vi "SS_observer_Delay.vi"(4 "Xd_in":T1=[0.0, 0.0, 0.0, 0.0, 0.0, 0.0, 0.0, 0.0, 0.0, 0.0, 0.0, 0.0] caption="Xd_In", 7 "y(k)":sgl format="%#_13g", 8 "Nd":u8, 9 "X":sgl[](array[numeric])=[0.0, 0.0, 0.0, 0.0, 0.0, 0.0, 0.0, 0.0, 0.0, 0.0, 0.0, 0.0, 0.0, 0.0, 0.0, 0.0, 0.0, 0.0, 0.0, 0.0, 0.0, 0.0, 0.0, 0.0, 0.0], 10 "u(predelay)(k)":sgl format="%#_13g", 11 "NS":i16) -> (3 "Ax + Bu + Lye":sgl[](array[numeric]), 6 "Xd_out":T1)   [LabVIEW 2017]
uses:
  controls/Xdelay.ctl
  <vilib>/Platform/TimedLoop/XDataNode/timing_clust.ctl
  <vilib>/Platform/TimedLoop/XDataNode/nitl_modes.ctl
  <vilib>/Platform/TimedLoop/XDataNode/wakeup.ctl
  <vilib>/rvi/Emulation/niFpgaSctlEmulationGetInTimedLoop.vi
  <vilib>/rvi/Emulation/niFpgaEmulationReportErrorSimple.vi
  <vilib>/rvi/Emulation/niFpgaGetClockAttributes.vi
  <vilib>/rvi/Emulation/niFpgaCriticalErrorInLSC.vi
  <vilib>/Platform/TimedLoop/XDataNode/XDataNode.xnode
  <vilib>/Platform/TimedLoop/XDataNode/XDNodeRunTimeDep.lvlib
panel:
  out "u(k)":sgl format="%#_13g"
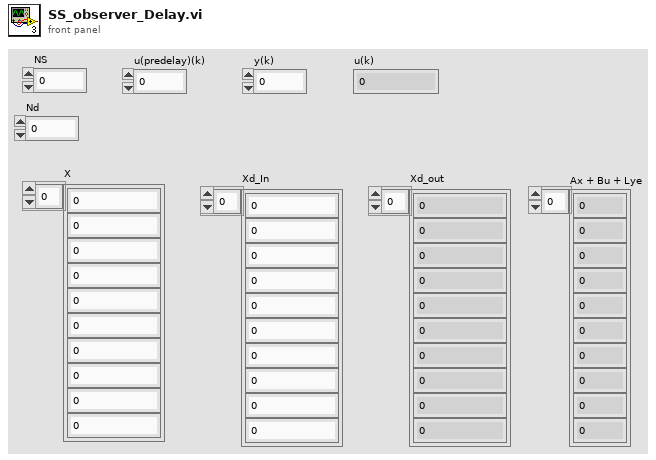
[diagram p1: front panel]
types:
  T1 = typedef "Xdelay.ctl" = sgl[]
  T2 = typedef "XDNodeRunTimeDep.lvlib/timing_clust.ctl" = cluster{"Expected End [f-1]":u64, "Actual End [f-1]":u64, "Finished Late? [f-1]":bool, "Expected End [i-1]":u64, "Actual End [i-1]":u64, "Finished Late? [i-1]":bool, "Expected Start [i]":u64, "Actual Start [i]":u64, "Expected Start [f]":u64, "Actual Start [f]":u64, "Source Name":string, "Structure Name":string, "Period":i64, "Deadline":i64, "Offset":i64, "Start":i64, "Priority":i32, "Timeout":i32, "Mode":T3, "Wakeup Reason":T4, "Error":errorcluster, "Source Type":string, "Secondary Source Type":string, "Global End Time":u64, "Global Start Time":u64, "Frame Duration":u64, "Iteration Duration":u64, "Assigned CPU":i32, "I/O Scan Engine Mode":u32}
  T3 = typedef "XDNodeRunTimeDep.lvlib/nitl_modes.ctl" = enum32{"No Change", "Process missed periods, maintain original phase", "Discard missed periods, maintain original phase", "Process missed periods, ignore original phase", "Discard missed periods, ignore original phase"}
  T4 = typedef "XDNodeRunTimeDep.lvlib/wakeup.ctl" = enum32{"Normal", "Aborted", "Asynchronous wakeup", "Timing source error", "Timed loop error", "Timeout"}
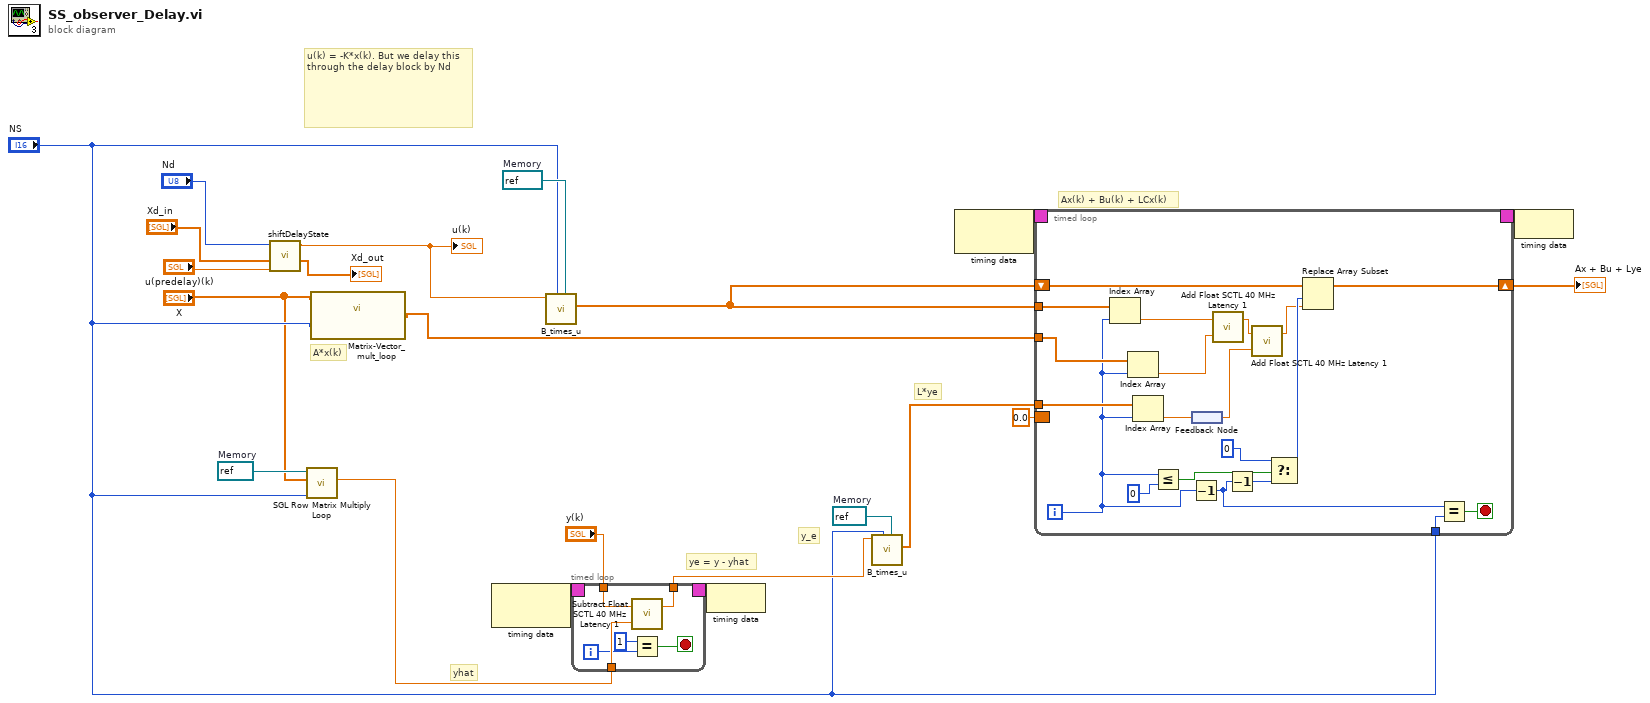
[diagram p0: block diagram]
diagram:
  w16 = refnum<k21> "L"  # Memory
  w15 = refnum<k21> "C"  # Memory
  w14 = refnum<k21> "Bz"  # Memory
  # "ye = y - yhat"
  # "yhat"
  # "A*x(k)"
  # "L*ye"
  # "y_e"
  # "u(k) = -K*x(k). But we delay this through the delay block by Nd"
  # "Ax(k) + Bu(k) + LCx(k)"
  n1 = call "shiftDelayState.vi"("u(k)"="u(predelay)(k)", "Xd_in"="Xd_in", "Nd"="Nd") -> ("Xd_out"=→"Xd_out":T1, "yd=C*Xd(k)"=w8:sgl)  [unwired: 7 in]
  "u(k)" <- w8
  n2 = call "SGL Row Matrix Multiply Loop.vi"("NS"="NS", "X"="X", "Refnum in"=w15) -> ("Numeric"=w12:sgl)  [unwired: 8 in]
  n3 = call "Matrix-Vector_mult_loop.vi"("Ns"="NS", "X"="X") -> ("A x X"=w3:sgl[])  [unwired: 9 in]
  n4 = node-c288() -> (w20:T2)  [unwired: 1 in]
  n5 = call "B_times_u.vi"("Memory"=w14, "NS"="NS", "u"=w8) -> ("product(vector)"=w9:sgl[])  [unwired: 8 in]
  n6 = timed-loop {
    timing: w20 -> [_]
    timing-out: [_] -> w19
    tunnel: [w28] -> w10
    tunnel: "y(k)" -> [w27]
    tunnel: w12 -> [w26]
    i -> [w24]
    stop <- w25 stop-if-true
    n7 = call "Subtract Float SCTL 40 MHz Latency 1.vi"("y"=w26, "x"=w27) -> ("x[k-1]-y[k-1]"=w28:sgl)  [unwired: 1 out]
    n8 = Equal?(x=i16 1, y=w24) -> (x = y?=w25:bool)
  }
  n9 = node-c288(w19) -> ()
  n10 = call "B_times_u.vi"("Memory"=w16, "NS"="NS", "u"=w10) -> ("product(vector)"=w11:sgl[])  [unwired: 8 in]
  n11 = node-c288() -> (w22:T2)  [unwired: 1 in]
  n12 = timed-loop {
    timing: w22 -> [_]
    timing-out: [_] -> w21
    tunnel: w9 -> [w48]
    tunnel: w3 -> [w49]
    tunnel: "NS" -> [w44]
    shift-right: [w47] -> w13
    shift-left: w9 -> [w46]
    tunnel: w11 -> [w41]
    border: sgl 0.0 -> [_]
    i -> [w37]
    stop <- w50 stop-if-true
    n13 = Index Array(array=w48, index=w37) -> (element=w43:sgl)
    n14 = Index Array(array=w49, index=w37) -> (element=w42:sgl)
    n15 = Index Array(array=w41, index=w37) -> (element=w39:sgl)
    n16 = Less Or Equal?(x=w37, y=i16 0) -> (x <= y?=w36:bool)
    n17 = Decrement(x=w37) -> (x-1=w32:i32)
    n18 = feedback #1() -> (w35:sgl)
    n19 = feedback-in #1(w39) -> ()
    n20 = call "Add Float SCTL 40 MHz Latency 1.vi"("y"=w42, "x"=w43) -> ("x[k-1]+y[k-1]"=w34:sgl)  [unwired: 1 out]
    n21 = Decrement(x=w32) -> (x-1=w31:i32)
    n22 = call "Add Float SCTL 40 MHz Latency 1.vi"("y"=w35, "x"=w34) -> ("x[k-1]+y[k-1]"=w33:sgl)  [unwired: 1 out]
    n23 = Select(t=i16 0, s=w36, f=w31) -> (s? t:f=w45:i32)
    n24 = Replace Array Subset(array=w46, new element=w33, index=w45) -> (w47:sgl[])
    n25 = Equal?(x=w32, y=w44) -> (x = y?=w50:bool)
  }
  "Ax + Bu + Lye" <- w13
  n26 = node-c288(w21) -> ()
